vi "Preset LOT NUMBER.vi"(8 "error in (no error)":errorcluster, 10 "LOT number":string, 11 "VISA resource in":refnum<visa-resource-name>) -> (0 "error out":errorcluster, 3 "VISA resource out":refnum<visa-resource-name>)   [LabVIEW 2025]
uses:
  lot number states--enum.ctl
  <instrlib>/Chroma 19052/Chroma 19052.lvlib
panel:
  # "Min 1 char, Max 13 char"
  # "Set LOT number"
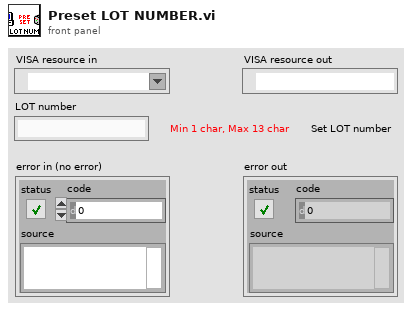
[diagram p1: front panel]
types:
  T1 = typedef "lot number states--enum.ctl" = enum16{"Initialize", "Check <=UL", "Check >=LL", "Truncate string", "Send command", "Shutdown"}
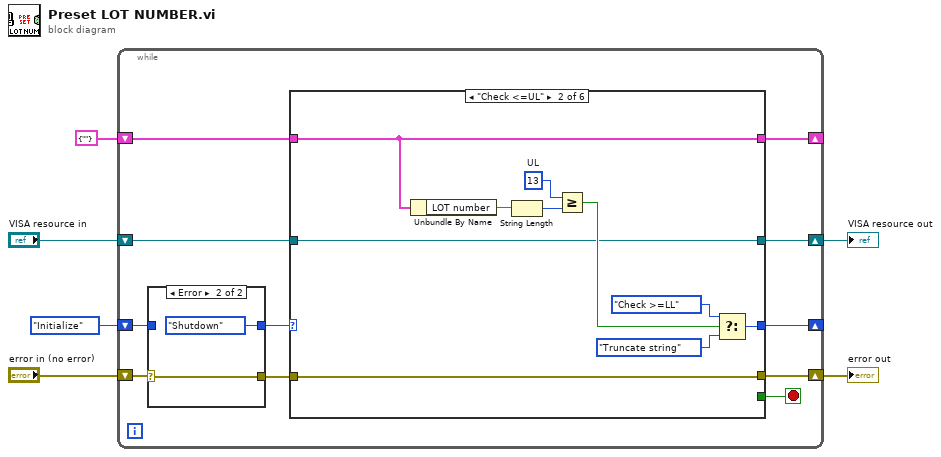
[diagram p0: block diagram]
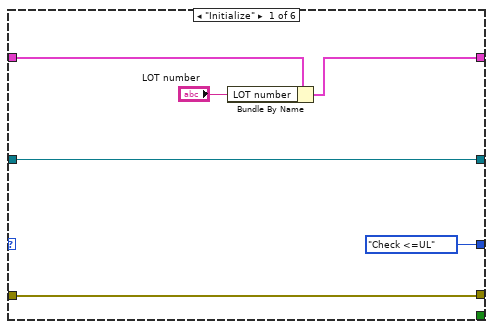
[diagram p3: hidden frame]
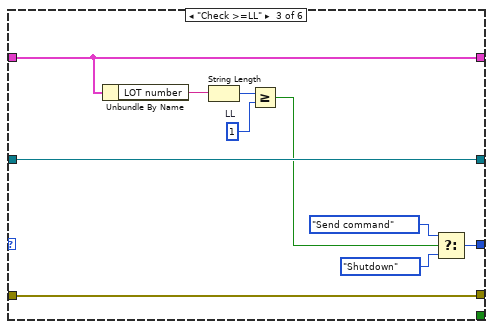
[diagram p4: hidden frame]
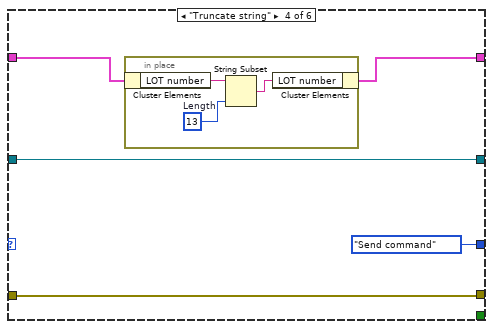
[diagram p5: hidden frame]
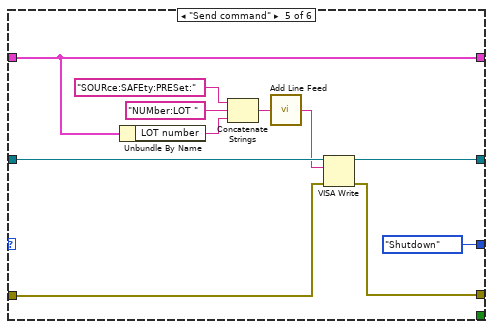
[diagram p6: hidden frame]
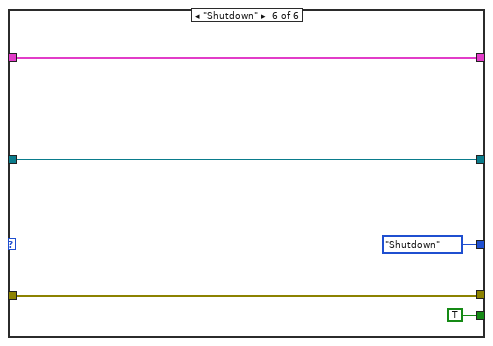
[diagram p7: hidden frame]
diagram:
  n1 = while {
    shift-right: [w14] -> _
    shift-left: lot_number_states--enum."Initialize" -> [w13]
    shift-right: [w8] -> _
    shift-left: cluster{"LOT number":string} {"LOT number"=""} -> [w15]
    shift-right: [w9] -> w3
    shift-left: "VISA resource in" -> [w12]
    shift-right: [w10] -> w4
    shift-left: "error in (no error)" -> [w16]
    stop <- w7 stop-if-true
    n2 = case shown="Error" w16 {
      selector: w16 -> [w19 w20]
      tunnel: [w19 w20] -> w11
      tunnel: [w18 lot_number_states--enum."Shutdown"] -> w17
      tunnel: w13 -> [w18 _]
      frame No Error {
      }
      frame Error {
      }
    }
    n3 = case shown="\"Check <=UL\"" w17 {
      tunnel: w15 -> [w25 w31 w40 w50 w57 w69]
      tunnel: [lot_number_states--enum."Check <=UL" w34 w43 lot_number_states--enum."Send command" lot_number_states--enum."Shutdown" lot_number_states--enum."Shutdown"] -> w14
      tunnel: w12 -> [w26 w33 w47 w52 w66 w71]
      tunnel: w11 -> [w27 w32 w46 w51 w65 w70]
      tunnel: [w27 w32 w46 w51 w64 w70] -> w10
      tunnel: [w26 w33 w47 w52 w63 w71] -> w9
      tunnel: [w24 w31 w40 w49 w57 w69] -> w8
      tunnel: [_ _ _ _ _ TRUE] -> w7
      frame "Initialize" {
        n4 = Bundle By Name(cluster=w25, "LOT number"="LOT number") -> (w24:cluster{"LOT number":string})
      }
      frame "Check <=UL" {
        w37 = 13  # UL
        n5 = Unbundle By Name(w31) -> ("LOT number"=w30:string)
        n6 = String Length(string=w30) -> (length=w36:i32)
        n7 = Greater Or Equal?(x=w37, y=w36) -> (x >= y?=w35:bool)
        n8 = Select(t=lot_number_states--enum."Check >=LL", s=w35, f=lot_number_states--enum."Truncate string") -> (s? t:f=w34:T1)
      }
      frame "Check >=LL" {
        w44 = 1  # LL
        n9 = Unbundle By Name(w40) -> ("LOT number"=w39:string)
        n10 = String Length(string=w39) -> (length=w45:i32)
        n11 = Greater Or Equal?(x=w45, y=w44) -> (x >= y?=w42:bool)
        n12 = Select(t=lot_number_states--enum."Send command" ("f"), s=w42, f=lot_number_states--enum."Shutdown") -> (s? t:f=w43:T1)
      }
      frame "Truncate string" {
        n13 = in-place {
          w54 = 13  # Length
          n14 = in-place-cluster #1(w50) -> ("LOT number"=w55:string)
          n15 = String Subset(string=w55, length (rest)=w54) -> (substring=w53:string)  [unwired: 1 in]
          n16 = in-place-cluster #1("LOT number"=w53) -> (w49:cluster{"LOT number":string})
        }
      }
      frame "Send command" {
        n17 = Unbundle By Name(w57) -> ("LOT number"=w56:string)
        n18 = Concatenate Strings("SOURce:SAFEty:PRESet:", "NUMber:LOT ", w56) -> (w59:string)
        n19 = call <instrlib>:"Add Line Feed.vi"("Command string"=w59) -> ("Concatenated string"=w58:string)  [unwired: 4 in]
        n20 = VISA Write(VISA resource name=w66, write buffer=w58, error in (no error)=w65) -> (VISA resource name out=w63:refnum<visa-resource-name>, error out=w64:errorcluster)  [unwired: 1 out]
      }
      frame "Shutdown" {
      }
    }
  }
  "error out" <- w4
  "VISA resource out" <- w3
